vi "PH_Cont-601k_PSU.get i attribute.vi"(0 "i ref in":refnum<vi>, 5 "error in (no error)":errorcluster) -> (14 "i ref out":refnum<vi>, 16 "i attribute":T1={"GUI Refs"={"Power On"=refnum, "Hard- and Software"=refnum, "Device Status"=refnum, "Device Error"=refnum, "Configuration"=refnum, "Flash Interval [s]"=refnum, "Interlock"=refnum, "Interlock Indicator"=refnum, "Voltage [V]"=refnum, "Readyness"=refnum, "Mode"=refnum, "Reset Error"=refnum, "Expert working"=refnum, "Charge"=refnum, "PSU On"=refnum}, "Interlock"=FALSE, "Service ID applied Voltage"=-1, "Device Settings"={"Configuration"=6, "Flash Interval [s]"=30.0, "Mode"=enum."STOP", "Voltage [V]"=0, "Charge"=FALSE, "VISA resource name"="COM1"}, "Readyness"={"Program"=enum."OFF", "Device"=enum."OFF"}, "Information"={"VISA resource name"="COM1", "Tagname Power On"="", "Interlock"={"Instance"="", "Tagname"=""}, "Limits [V]"={"Lower"=0.0, "Upper"=0.0}, "Tagname PSU On"=""}, "R2S"=FALSE, "Charge is allowed"=FALSE} {"Device Settings"."Voltage [V]" max=2000 step=10; "Device Settings"."Flash Interval [s]" min=5.0 max=60.0 step=1.0; "Device Settings"."Configuration" items=["Ch intl, Fl intl, QSw intl", "Ch intl, Fl intl, QSw ext", "Ch intl, Fl ext, QSw intl", "Ch intl, Fl ext, QSw ext", "Ch ext, Fl int, QSw int", "Ch ext, Fl int, QSw ext", "Ch ext, Fl ext, QSw int", "Ch ext, Fl ext, QSw ext"]}, 19 "error out":errorcluster)   [LabVIEW 2014, in "PH_Cont-601k_PSU.lvlib"]
doc: "Gets the i attribute data of an object.\n\nLicense Agreement for this software:\n\nCopyright (C)\nGesellschaft für Schwerionenforschung, GSI\nPlanckstr. 1\n64291 Darmstadt\nGermany\n\nContact: D.Beck@gsi.de \n\nThis program is free software; you can redistribute it and/or modify it under the terms of the GNU General Public License as published by the Free Software Foundation; either version 2 of the license, or (at your option) any later version.\n\nThis program is distributed in the hope that it will be useful, but WITHOUT ANY WARRANTY; without even the implied warranty of MERCHANTABILITY or FITNESS FOR A PARTICULAR PURPOSE. See the GNU General License for more details (http://www.gnu.org).\n\nGesellschaft für Schwerionenforschung, GSI\nPlanckstr. 1, 64291 Darmstadt, Germany\nFor all questions and ideas contact: M.Richter@gsi.de, H.Brand@gsi.de or D.Beck@gsi.de.\nLast update: 17-JUN-2004"
uses:
  PH_Cont-601k_PSU.lvlib
  PH_Cont-601k_PSU.i attribute.ctl
  PH_Cont-601k_PSU.GUI Refs.ctl
  PH_Cont-601k_PSU.Device Status.ctl
  PH_Cont-601k_PSU.Readyness.ctl
  PH_Cont-601k_PSU.Readyness Program.ctl
  PH_Cont-601k_PSU.Readyness Device.ctl
  PH_Cont-601k_PSU.Mode.ctl
  PH_Cont-601k_PSU.Configuration.ctl
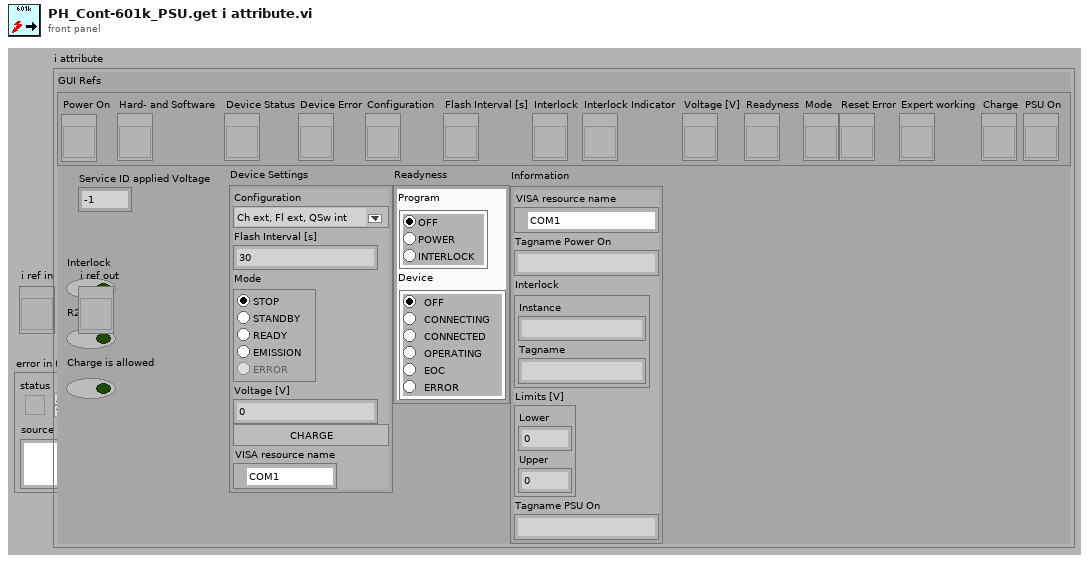
[diagram p1: front panel]
types:
  T1 = typedef "PH_Cont-601k_PSU.lvlib/PH_Cont-601k_PSU.i attribute.ctl" = cluster{"GUI Refs":T2, "Interlock":bool, "Service ID applied Voltage":i32, "Device Settings":cluster{"Configuration":T3, "Flash Interval [s]":dbl, "Mode":T4, "Voltage [V]":u16, "Charge":bool, "VISA resource name":refnum<visa-resource-name>}, "Readyness":T5, "Information":cluster{"VISA resource name":refnum<visa-resource-name>, "Tagname Power On":string, "Interlock":cluster{"Instance":string, "Tagname":string}, "Limits [V]":cluster{"Lower":dbl, "Upper":dbl}, "Tagname PSU On":string}, "R2S":bool, "Charge is allowed":bool}
  T2 = typedef "PH_Cont-601k_PSU.lvlib/PH_Cont-601k_PSU.GUI Refs.ctl" = cluster{"Power On":refnum<vi>, "Hard- and Software":refnum<vi>, "Device Status":refnum<vi>, "Device Error":refnum<vi>, "Configuration":refnum<vi>, "Flash Interval [s]":refnum<vi>, "Interlock":refnum<vi>, "Interlock Indicator":refnum<vi>, "Voltage [V]":refnum<vi>, "Readyness":refnum<vi>, "Mode":refnum<vi>, "Reset Error":refnum<vi>, "Expert working":refnum<vi>, "Charge":refnum<vi>, "PSU On":refnum<vi>}
  T3 = typedef "PH_Cont-601k_PSU.lvlib/PH_Cont-601k_PSU.Configuration.ctl" = u16
  T4 = typedef "PH_Cont-601k_PSU.lvlib/PH_Cont-601k_PSU.Mode.ctl" = enum32{"STOP", "STANDBY", "READY", "EMISSION", "ERROR"}
  T5 = typedef "PH_Cont-601k_PSU.lvlib/PH_Cont-601k_PSU.Readyness.ctl" = cluster{"Program":T6, "Device":T7}
  T6 = typedef "PH_Cont-601k_PSU.lvlib/PH_Cont-601k_PSU.Readyness Program.ctl" = enum32{"OFF", "POWER", "INTERLOCK"}
  T7 = typedef "PH_Cont-601k_PSU.lvlib/PH_Cont-601k_PSU.Readyness Device.ctl" = enum32{"OFF", "CONNECTING", "CONNECTED", "OPERATING", "EOC", "ERROR"}
  T8 = enum16{"SetAttribute", "GetAttribute", "CreateAttribute", "DestroyAttribute", "DestroyAllAtributes"}
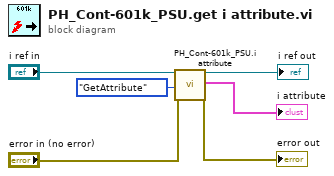
[diagram p0: block diagram]
diagram:
  n1 = call "PH_Cont-601k_PSU.i attribute.vi"("VI Refnum"="i ref in", "Action"=T8."GetAttribute", "error in (no error)"="error in (no error)") -> ("VI Refnum out"=→"i ref out":refnum<vi>, "CLASS.i attribute out"=→"i attribute":T1, "error out"=→"error out":errorcluster)  [unwired: 14 in]
